vi "Actor Core.vi"(8 "error in":errorcluster, 11 "Bob in":refnum<class "Bob.lvclass">) -> (0 "error out":errorcluster, 3 "Bob out":refnum<class "Actor.lvclass">)   [LabVIEW 2014, in "Bob.lvlib" / "Bob.lvclass"]
doc: "(<B>Filename</B>: Actor Framework.lvlib:Actor.lvclass:Actor Core.vi)\n\nReceives messages to the actor, reacts to them, and initiates any error handling that may shut the actor down.\n\nDescendant classes may override this VI to append parallel tasks for the actor to complete while it handles messages. Overrides use the Call Parent Method node."
uses:
  Bob.lvclass
  <vilib>/ActorFramework/Actor/Actor.lvclass
  <vilib>/ActorFramework/Actor/Actor.lvclass/Actor.ctl
  <vilib>/ActorFramework/Message Enqueuer/Message Enqueuer.lvclass/Message Enqueuer.ctl
  <vilib>/ActorFramework/Message Enqueuer/Init from Existing Queue.vi
  <vilib>/ActorFramework/Message Enqueuer/Enqueue.vi
  <vilib>/ActorFramework/Message Priority Queue/Priority Enqueue.vi
  <vilib>/ActorFramework/Message Enqueuer/Message Enqueuer.lvclass
  <vilib>/ActorFramework/Stop Msg/Stop Msg.lvclass
  Bob Messages/Send to Alice Msg/Send to Alice Msg.lvclass
panel:
  in  "stop 2":bool
  in  "stop":bool
  in  "Send to Alice":bool
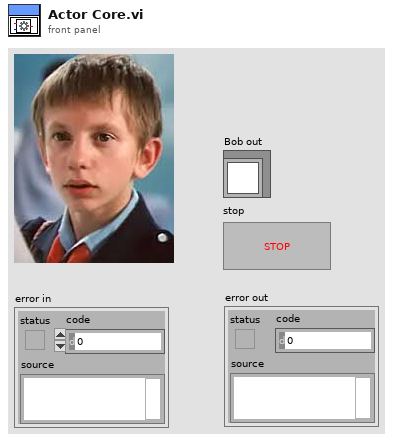
[diagram p1: front panel]
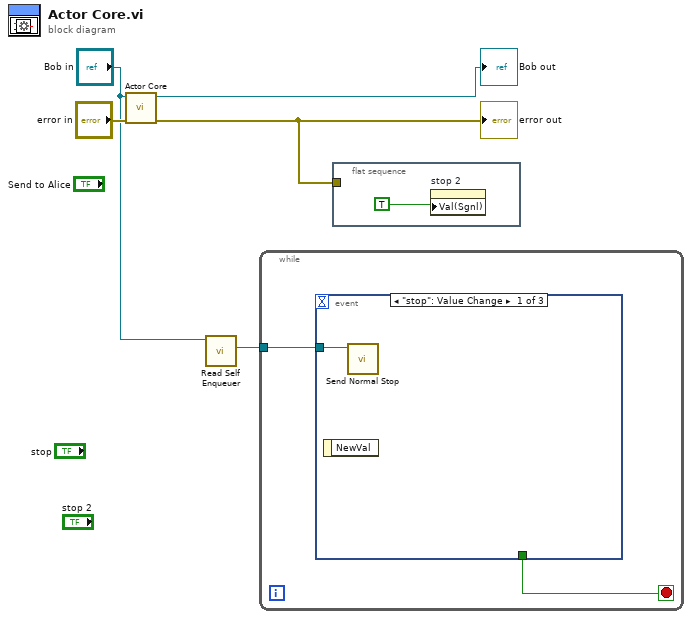
[diagram p0: block diagram]
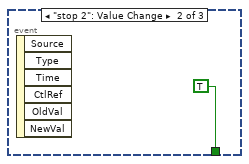
[diagram p2: hidden frame]
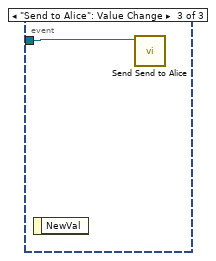
[diagram p3: hidden frame]
diagram:
  n1 = call-parent "Actor Core.vi"("error in"="error in", "Actor in"="Bob in") -> ("error out"=w2:errorcluster, "Actor out"=→"Bob out":refnum<class "Actor.lvclass">)  [unwired: 8 in]
  "error out" <- w2
  n2 = call <vilib>:"Read Self Enqueuer.vi"("Actor"="Bob in") -> ("Self Enqueuer"=w3:refnum<class "Message Enqueuer.lvclass">)  [unwired: 10 in]
  n3 = while {
    tunnel: w3 -> [w7]
    stop <- w6 stop-if-true
    n4 = event shown="[0] \"stop\": Value Change" {
      selector: _ -> [_ _ _]
      dyn-events: _ -> [_ _ _]
      timeout: _ -> [_ _ _]
      tunnel: w7 -> [w8 _ w10]
      tunnel: [_ TRUE _] -> w6
      event "stop": Value Change {
        n5 = event-data() -> ()  [unwired: 1 in, 1 out]
        n6 = call <vilib>:"Send Normal Stop.vi"("Message Enqueuer"=w8) -> ()  [unwired: 10 in, 1 out]
      }
      event "stop 2": Value Change {
        n7 = event-data() -> ()  [unwired: 1 in, 6 out]
      }
      event "Send to Alice": Value Change {
        n8 = event-data() -> ()  [unwired: 1 in, 1 out]
        n9 = call "Send Send to Alice.vi"("Message Enqueuer"=w10) -> ()  [unwired: 9 in, 2 out]
      }
    }
  }
  n10 = flat-sequence {
    tunnel: w2 -> [_]
    frame #0 {
      n11 = property on="stop 2" class="Bool (strict)"("Val(Sgnl)"=TRUE) -> ()  [unwired: 2 in, 2 out]
    }
  }
